vi "Global 1.vi"() -> ()   [LabVIEW 2025]
panel:
  in  "UserLevel":string
  in  "Logged user":string
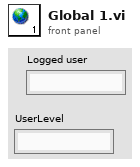
[diagram p1: front panel]
diagram:
